vi "Convert I32 to SGL-host.vi"(7 "Input":i32) -> (8 "Output SGL":sgl)   [LabVIEW 2011]
uses:
  <vilib>/rvi/FXPMathLib/FxpInterpret/XNode/nifxpmath_Interpret.xnode
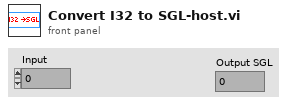
[diagram p1: front panel]
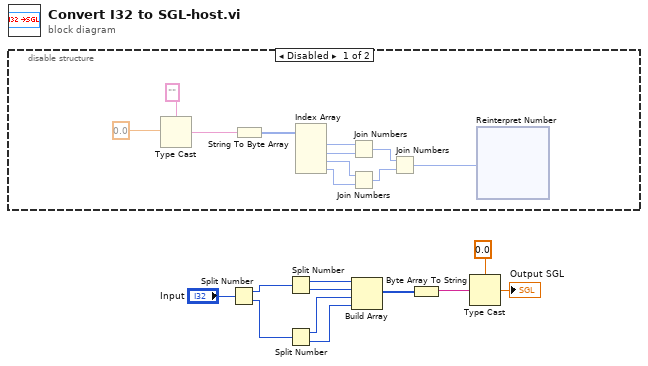
[diagram p0: block diagram]
diagram:
  n1 = disable-structure shown="Disabled" {
    frame Disabled {
      n2 = Type Cast(type="", x=sgl 0.0 ("Input")) -> (*(type *) &x=w21:string)
      n3 = String To Byte Array(string=w21) -> (unsigned byte array=w20:u8[])
      n4 = Index Array(array=w20) -> (element #1=w18:u8, element #2=w19:u8, element #3=w17:u8, element #4=w16:u8)  [unwired: 4 in]
      n5 = Join Numbers(hi=w18, lo=w19) -> ((hi.lo)=w14:u16)
      n6 = Join Numbers(hi=w17, lo=w16) -> ((hi.lo)=w15:u16)
      n7 = Join Numbers(hi=w14, lo=w15) -> ((hi.lo)=w13:u32)
      n8 = xnode "Reinterpret Number"("x"=w13) -> ()  [unwired: 1 out]
    }
    frame Enabled {
    }
  }
  n9 = Split Number(x="Input") -> (hi(x)=w11:u16, lo(x)=w10:u16)
  n10 = Split Number(x=w11) -> (hi(x)=w9:u8, lo(x)=w8:u8)
  n11 = Split Number(x=w10) -> (hi(x)=w7:u8, lo(x)=w6:u8)
  n12 = Build Array(w9, w8, w7, w6) -> (w5:u8[])
  n13 = Byte Array To String(unsigned byte array=w5) -> (string=w4:string)
  n14 = Type Cast(type=sgl 0.0 ("Input"), x=w4) -> (*(type *) &x=→"Output SGL":sgl)
